vi "Soln.vi"(1 "Celsius":dbl) -> (0 "Fahrenheit":dbl)   [LabVIEW 2017]
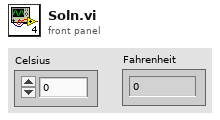
[diagram p1: front panel]
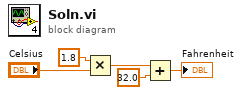
[diagram p0: block diagram]
diagram:
  n1 = Multiply(x=1.8, y="Celsius") -> (x*y=w3:dbl)
  n2 = Add(x=w3, y=32.0) -> (x+y=→"Fahrenheit":dbl)
